vi "calculate_segment_sections.vi"(8 "error in":errorcluster, 9 "range (m)":dbl, 10 "Angle WP to second leyline (deg)":dbl, 11 "Angle WP to first leyline (deg)":dbl) -> (0 "error out":errorcluster, 1 "Angle between leylines (deg)":dbl, 2 "Length of second leg (m)":dbl, 3 "Length of first leg (m)":dbl)   [LabVIEW 2013]
doc: "This VI takes the absolute angle difference between (boat-waypoint) and (boat-leyline) for both leylines, as well as the range of the tack.\n\nIf you imagine the two leylines being 45 degrees off of the (boat-waypoint) line, that would mean the boat is tacking directly upwind. This function returns the side lengths of a triangle where the given range is the longest leg.\n\nEric Schneider, September 2014\n\n a2 | \\ L2\n | \\\nrange | /\n | /\n a1 | / L1\n |/"
uses:
  <vilib>/imath/engines/lvmath2/RunTimeEngine/ErrorHandling/NIMS_Finalize Error.vi
  <vilib>/imath/engines/lvmath2/RunTimeEngine/Managers/WorkSpace/UID Generator.vi
  <vilib>/imath/engines/lvmath2/RunTimeEngine/Managers/SymbolTable/Clear UID.vi
  <vilib>/imath/engines/lvmath2/RunTimeEngine/NodeEndStatement/NIMS_NodeEndStatement_Output.vi
  <instcachedir>/0/NIMS_NodeEndStatement_Output_53EC0D466D134D7ABD903AC30B43404B.lvgen/NIMS_NodeEndStatement_Output_53EC0D466D134D7ABD903AC30B43404B_001.vi
  <vilib>/imath/engines/lvmath2/RunTimeEngine/RunTimeType/NIMS_RunTimeType_From StrictType (excl LVString).vi
  <instcachedir>/0/NIMS_RunTimeType_From StrictType (excl LVString)_4DEE718D6EB74582AA20236969C084FC.lvgen/NIMS_RunTimeType_From StrictType (excl LVString)_4DEE718D6EB74582AA20236969C084FC_000.vi
  <vilib>/imath/engines/lvmath2/RunTimeEngine/LocalVariableDefStatement/MC_LocalVariableDefStatement_Display.vi
  <vilib>/imath/engines/lvmath2/RunTimeEngine/Managers/SymbolTable/NIMS_WorkSpace.lvlib
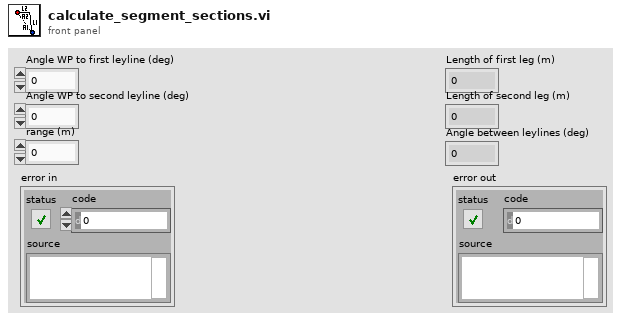
[diagram p1: front panel]
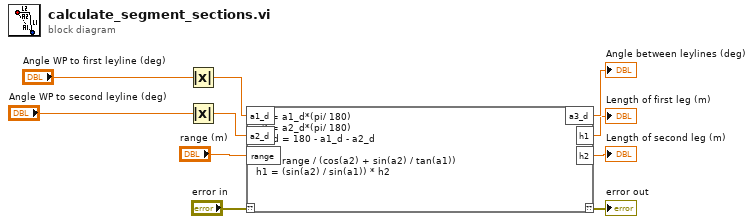
[diagram p0: block diagram]
diagram:
  n1 = Absolute Value(x="Angle WP to first leyline (deg)") -> (abs(x)=w1:dbl)
  n2 = Absolute Value(x="Angle WP to second leyline (deg)") -> (abs(x)=w3:dbl)
  n3 = mathscript code="a1 = a1_d*(pi/ 180)\na2 = a2_d*(pi/ 180)\na3_d = 180 - a1_d - a2_d\n\nh2 = range / (cos(a2) + sin(a2) / tan(a1))\nh1 = (sin(a2) / sin(a1)) * h2"("??"="error in", "range"="range (m)", "a1_d"=w1, "a2_d"=w3) -> ("??"=→"error out":errorcluster, "a3_d"=→"Angle between leylines (deg)":dbl, "h1"=→"Length of first leg (m)":dbl, "h2"=→"Length of second leg (m)":dbl)
